vi "niRFUtil CAL Retrieve Calibration Data.vi"(0 "Calibration Path Name":T4="dut_to_vsa", 11 "error in (no error)":errorcluster, 12 "Folder Path":T1) -> (6 "Calibration Data":T2 {"Calibration Table" min=0 max=127 format="%.2p"; "Time Stamp (sec)" format="%^.2e"; "Temperature (C)" format="%.1f"}, 15 "error out":errorcluster)   [LabVIEW 2015, in "niRFUtil.lvlib"]
doc: "This utility retrieves the calibration data from an .tdms file. \nString name get converted to a file path relative to the VIs path.\n\n(c) Copyright 2006, National Instruments, Inc. This VI may not be duplicated, sold, or distributed without written consent from National Instruments."
uses:
  niRFUtil.lvlib
  Includes/niRFUtil INC Calibration Signal Path Name.ctl
  Includes/niRFUtil INC Calibration Data.ctl
  Includes/niRFUtil INC Calibration Table.ctl
  Includes/niRFUtil INC Calibration File Path Folder.ctl
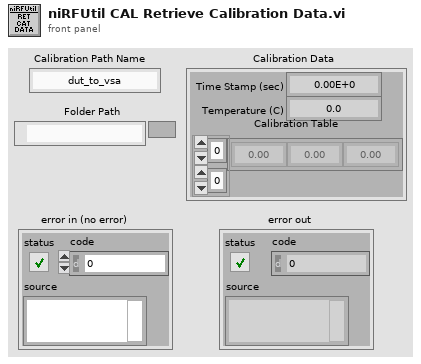
[diagram p1: front panel]
types:
  T1 = typedef "niRFUtil.lvlib/niRFUtil INC Calibration File Path Folder.ctl" = path
  T2 = typedef "niRFUtil.lvlib/niRFUtil INC Calibration Data.ctl" = cluster{"Temperature (C)":dbl, "Time Stamp (sec)":dbl, "Calibration Table":T3}
  T3 = typedef "niRFUtil.lvlib/niRFUtil INC Calibration Table.ctl" = sgl[][]
  T4 = typedef "niRFUtil.lvlib/niRFUtil INC Calibration Signal Path Name.ctl" = string
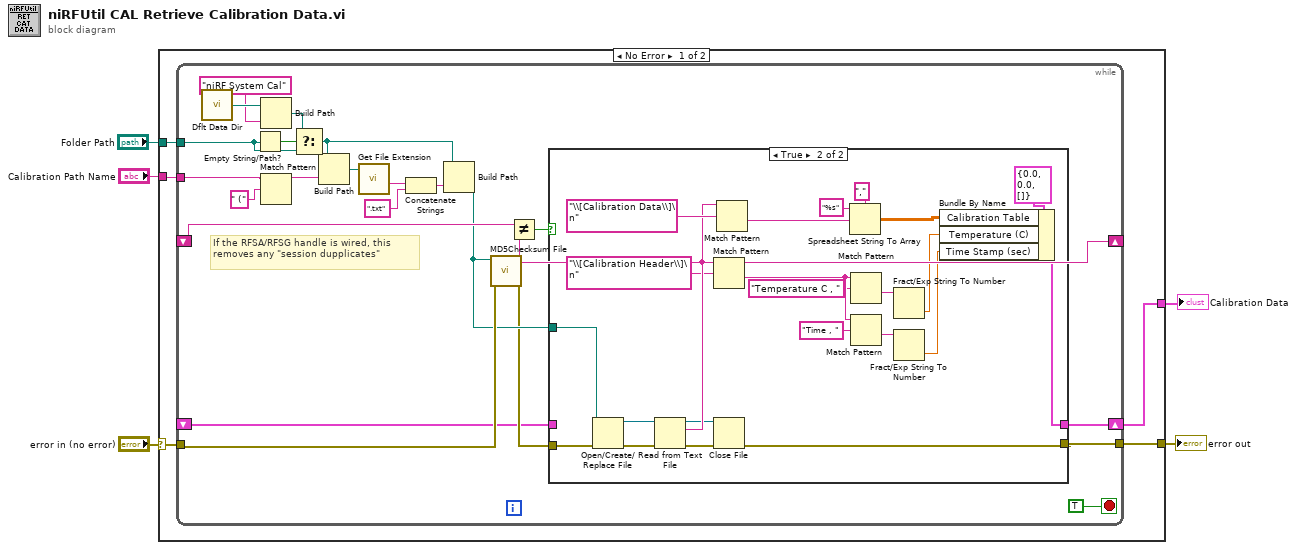
[diagram p0: block diagram]
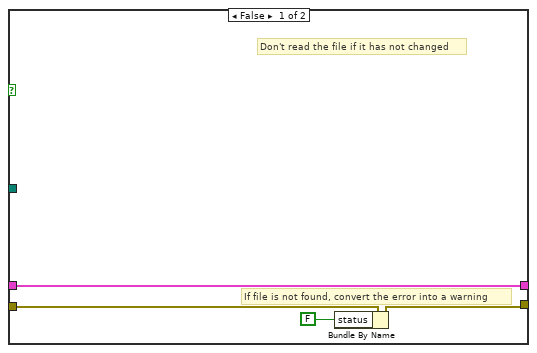
[diagram p2: hidden frame]
diagram:
  n1 = case shown="No Error" "error in (no error)" {
    selector: "error in (no error)" -> [w10 w61]
    tunnel: [w9 w61] -> w4
    tunnel: "Calibration Path Name" -> [w7 _]
    tunnel: [w8 _] -> w2
    tunnel: "Folder Path" -> [w6 _]
    frame No Error {
      n2 = while {
        tunnel: w10 -> [w31]
        tunnel: [w21] -> w9
        shift-right: [w11] -> _
        shift-left: _ -> [w32]
        tunnel: w7 -> [w16]
        shift-right: [w22] -> w8
        shift-left: _ -> [w23]
        tunnel: w6 -> [w19]
        stop <- TRUE stop-if-true
        # "If the RFSA/RFSG handle is wired, this removes any \"session dupplicates\""
        n3 = call <vilib>:"Dflt Data Dir.vi"() -> ("App:Default Data Directory"=w13:path)
        n4 = Empty String/Path?(string/path=w19) -> (empty?=w20:bool)
        n5 = Build Path(base path=w13, name or relative path="niRF System Cal") -> (appended path=w17:path)
        n6 = Match Pattern(string=w16, regular expression=" (") -> (before substring=w15:T4)  [unwired: 1 in, 3 out]
        n7 = Select(t=w17, s=w20, f=w19) -> (s? t:f=w18:T1)
        n8 = Build Path(base path=w18, name or relative path=w15) -> (appended path=w30:path)
        n9 = call <vilib>:"Get File Extension.vi"("file"=w30) -> ("filename without extension"=w29:string)  [unwired: 1 in, 9 out]
        n10 = Concatenate Strings(w29, ".txt" ("string")) -> (w27:string)
        n11 = Build Path(base path=w18, name or relative path=w27) -> (appended path=w25:path)
        n12 = call <vilib>:"MD5Checksum File.vi"("error in (no error)"=w31, "Path"=w25) -> ("error out"=w24:errorcluster, "MD5 message-digest"=w11:string)  [unwired: 8 out]
        n13 = Not Equal?(x=w32, y=w11) -> (x != y?=w26:bool)
        n14 = case shown="True" w26 {
          tunnel: [w35 w40] -> w21
          tunnel: w25 -> [_ w42]
          tunnel: w24 -> [w36 w41]
          tunnel: [w34 w39] -> w22
          tunnel: w23 -> [w34 _]
          frame False {
            # "If file is not found, convert the error into a warning"
            # "Don't read the file if it has not changed"
            n15 = Bundle By Name(cluster=w36, "status"=FALSE) -> (w35:errorcluster)
          }
          frame True {
            n16 = Open/Create/Replace File(file path (use dialog)=w42, error in=w41) -> (refnum out=w43:refnum<file>, error out=w44:errorcluster)  [unwired: 4 in, 1 out]
            n17 = Read from Text File(file (use dialog)=w43, error in=w44) -> (refnum out=w45:refnum<file>, text=w48:string, error out=w46:errorcluster)  [unwired: 2 in, 1 out]
            n18 = Match Pattern(string=w48, regular expression="\\[Calibration Header\\]\n") -> (after substring=w58:string)  [unwired: 1 in, 3 out]
            n19 = Close File(refnum=w45, error in=w46) -> (error out=w40:errorcluster)  [unwired: 1 out]
            n20 = Match Pattern(string=w48, regular expression="\\[Calibration Data\\]\n") -> (after substring=w50:string)  [unwired: 1 in, 3 out]
            n21 = Spreadsheet String To Array(delimiter (Tab)=",", format string="%s", spreadsheet string=w50) -> (array=w53:dbl[][])  [unwired: 1 in]
            n22 = Match Pattern(string=w58, regular expression="Temperature C , ") -> (after substring=w55:string)  [unwired: 1 in, 3 out]
            n23 = Match Pattern(string=w58, regular expression="Time , ") -> (after substring=w57:string)  [unwired: 1 in, 3 out]
            n24 = Fract/Exp String To Number(string=w55) -> (number=w56:dbl)  [unwired: 3 in, 1 out]
            n25 = Fract/Exp String To Number(string=w57) -> (number=w60:dbl)  [unwired: 3 in, 1 out]
            n26 = Bundle By Name(cluster=T2 {"Temperature (C)"=0.0, "Time Stamp (sec)"=0.0, "Calibration Table"=[]} ("Calibration Data 2"), "Calibration Table"=w53, "Temperature (C)"=w56, "Time Stamp (sec)"=w60) -> (w39:T2)
          }
        }
      }
    }
    frame Error {
    }
  }
  "error out" <- w4
  "Calibration Data" <- w2
